vi "Read Measurement Description Dictionary.vi"(8 "error in (no error)":errorcluster, 11 "NI Generic Parser in":refnum<class "NI Generic Parser.lvclass">) -> (0 "error out":errorcluster, 2 "NI Generic Parser.lvlib:Multi Step Database":refnum<class "Multi Step Database.lvclass">, 3 "NI Generic Parser out":refnum<class "NI Generic Parser.lvclass">)   [LabVIEW 2016, in "NI Generic Parser.lvlib" / "NI Generic Parser.lvclass"]
uses:
  NI Generic Parser.lvclass
  Support/Step Sequence Database/Multi Step Database.lvclass
  NI Generic Parser.lvclass/NI Generic Parser.ctl
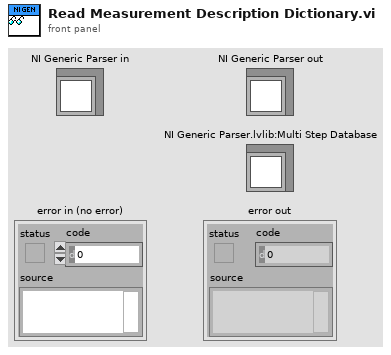
[diagram p1: front panel]
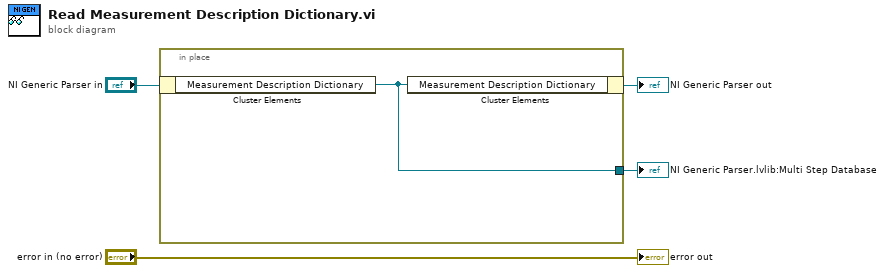
[diagram p0: block diagram]
diagram:
  n1 = in-place {
    in-place-border: [w5] -> w2
    n2 = in-place-cluster #1("NI Generic Parser in") -> ("Measurement Description Dictionary"=w5:refnum<class "Multi Step Database.lvclass">)
    n3 = in-place-cluster #1("Measurement Description Dictionary"=w5) -> (→"NI Generic Parser out":refnum<class "NI Generic Parser.lvclass">)
  }
  "NI Generic Parser.lvlib:Multi Step Database" <- w2
  "error out" <- "error in (no error)"
